vi "Read Dependencies.vi"(8 "error in (no error)":errorcluster, 11 "system in":refnum<class "system.lvclass">) -> (0 "error out":errorcluster, 2 "Dependencies":T1, 3 "system":refnum<class "system.lvclass">)   [LabVIEW 2016, in "system.lvclass"]
uses:
  system.lvclass
  Typedefs/Dependencies-cluster.ctl
  DAQ_Manager/DAQ_Manager.lvclass
  DSP/DSP.lvclass
  Generator/Generator.lvclass
  Scope/Scope.lvclass
  system.lvclass/system.ctl
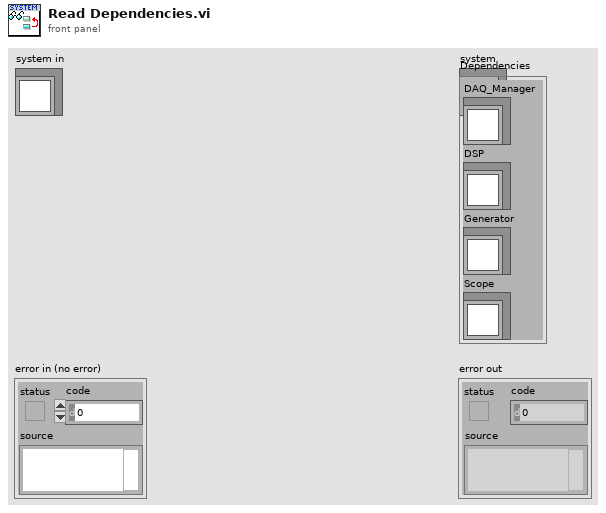
[diagram p1: front panel]
types:
  T1 = typedef "system.lvclass/Dependencies-cluster.ctl" = cluster{"DAQ_Manager":refnum<class "DAQ_Manager.lvclass">, "DSP":refnum<class "DSP.lvclass">, "Generator":refnum<class "Generator.lvclass">, "Scope":refnum<class "Scope.lvclass">}
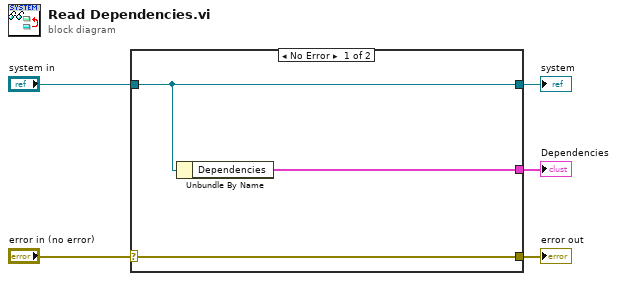
[diagram p0: block diagram]
diagram:
  n1 = case shown="No Error" "error in (no error)" {
    selector: "error in (no error)" -> [w8 w9]
    tunnel: [w8 w9] -> w4
    tunnel: [w7 w10] -> w2
    tunnel: "system in" -> [w7 w10]
    tunnel: [w6 _] -> w1
    frame No Error {
      n2 = Unbundle By Name(w7) -> ("Dependencies"=w6:T1)
    }
    frame Error {
    }
  }
  "error out" <- w4
  "system" <- w2
  "Dependencies" <- w1
